vi "Launch Nested AF.vi"(8 "error in (no error)":errorcluster, 9 "name":string, 10 "Nested Actor":refnum<class "Actor.lvclass">, 11 "[V] Main UI in":refnum<class "[V] Main UI.lvclass">) -> (0 "error out":errorcluster, 2 "Enqueuer":refnum<class "Message Enqueuer.lvclass">, 3 "[V] Main UI out":refnum<class "[V] Main UI.lvclass">)   [LabVIEW 2020, in "[V] Main UI.lvlib" / "[V] Main UI.lvclass"]
uses:
  [V] Main UI.lvclass
  <vilib>/ActorFramework/Actor/Actor.lvclass
  <vilib>/ActorFramework/Message Enqueuer/Message Enqueuer.lvclass
  Depden On/MVVM Framework/MVVM Abstruct View/MVVM Abstruct View/Accessor/Read ActorMap-Views.vi
  Depden On/ActorMap/ActorMap.lvclass
  Depden On/MVVM Framework/MVVM Abstruct View/MVVM Abstruct View/MVVM Abstruct View.lvclass
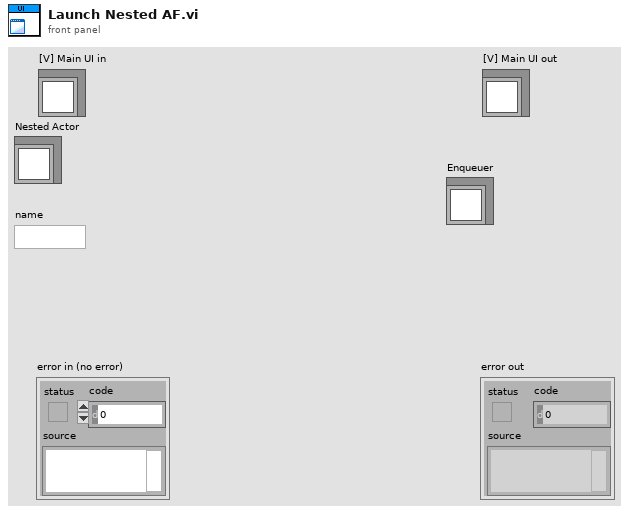
[diagram p1: front panel]
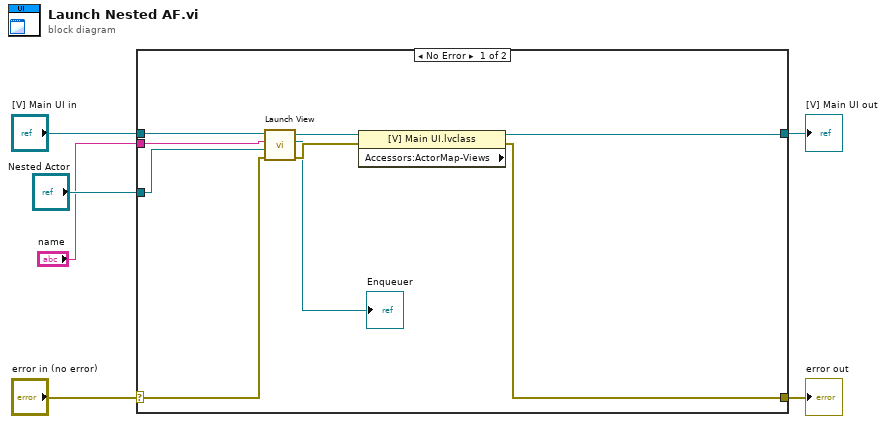
[diagram p0: block diagram]
diagram:
  n1 = case shown="No Error" "error in (no error)" {
    selector: "error in (no error)" -> [w10 w17]
    tunnel: [w7 w17] -> w5
    tunnel: [w9 w16] -> w3
    tunnel: "[V] Main UI in" -> [w15 w16]
    tunnel: "Nested Actor" -> [w14 _]
    tunnel: "name" -> [w13 _]
    frame No Error {
      n2 = call "Launch View.vi"("error in (no error)"=w10, "Actor"=w14, "Name"=w13, "MVVM Abstruct View in"=w15) -> ("error out"=w11:errorcluster, "Nested Actor's Enqueuer"=→"Enqueuer":refnum<class "Message Enqueuer.lvclass">, "MVVM Abstruct View out"=w12:refnum<class "[V] Main UI.lvclass">)  [unwired: 5 in]
      n3 = property class="[V] Main UI.lvclass" props=["Accessors:ActorMap-Views"](reference=w12, error in=w11) -> (reference out=w9:refnum<class "[V] Main UI.lvclass">, error out=w7:errorcluster)  [unwired: 1 out]
    }
    frame Error {
    }
  }
  "error out" <- w5
  "[V] Main UI out" <- w3
